vi "Cleanup Session.vi"(8 "error in":errorcluster, 11 "Plugin in":refnum<class "Power Spectrum Density.lvclass">) -> (0 "error out":errorcluster, 3 "Plugin out":refnum<class "Power Spectrum Density.lvclass">)   [LabVIEW 2023, in "Power Spectrum Density.lvlib" / "Power Spectrum Density.lvclass"]
uses:
  Power Spectrum Density.lvclass
  Buffer Manager Function.ctl
  Power Spectrum Density.lvclass/Power Spectrum Density.ctl
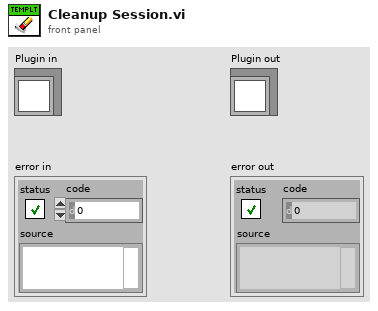
[diagram p1: front panel]
types:
  T1 = typedef "Power Spectrum Density.lvlib/Power Spectrum Density.lvclass/Buffer Manager Function.ctl" = enum16{"Get Data", "Buffer Data", "Reset Data"}
  T2 = enum32{"Invalid", "Standard", "Closed", "Hidden", "Minimized", "Maximized"}
  T3 = typedef "Power Spectrum Density.lvlib/Power Spectrum Density.lvclass/Power Spectrum Density Data.ctl" = cluster{"First Time":bool, "Show PSD Window":bool, "Show PSD Window Clicked":bool, "Export mode":T4, "Window":T5, "dB":bool, "Averaging parameters":cluster{"averaging mode":enum16{"No averaging", "Vector averaging", "RMS averaging", "Peak hold"}, "weighting mode":enum16{"Linear", "Exponential"}, "number of averages":u32}, "Window parameter":dbl, "Number of Samples":i32, "PSD VI Ref":refnum<vi>}
  T4 = typedef "NI_MAPro.lvlib/Power Spectrum and PSD Export Mode.ctl" = u16
  T5 = typedef "NI_AALPro.lvlib/windowTd.ctl" = u32
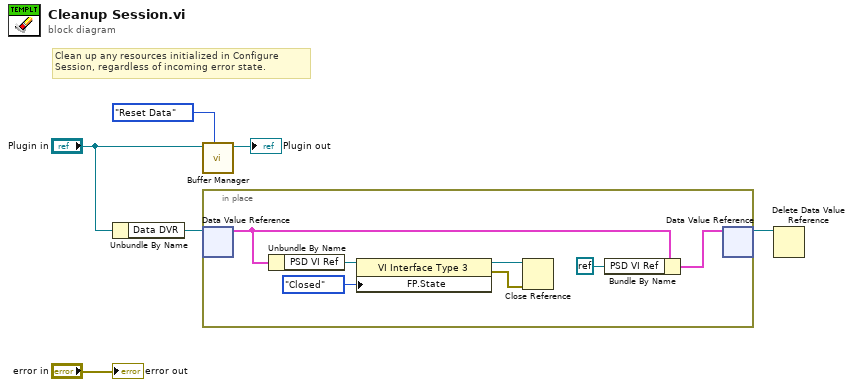
[diagram p0: block diagram]
diagram:
  # "Clean up any resources initialized in Configure Session, regardless of incoming error state."
  n1 = Unbundle By Name("Plugin in") -> ("Data DVR"=w6:refnum<data-value>)
  n2 = call-dynamic "Buffer Manager.vi"("Function"=Buffer_Manager_Function."Reset Data", "Plugin in"="Plugin in") -> ("Plugin out"=→"Plugin out":refnum<class "Power Spectrum Density.lvclass">)  [unwired: 5 in, 4 out]
  n3 = in-place {
    n4 = in-place-dvr #1(w6) -> (w13:T3)  [unwired: 1 out]
    n5 = Unbundle By Name(w13) -> ("PSD VI Ref"=w10:refnum<vi>)
    n6 = property class="VI Interface Type 3"(reference=w10, "FP.State"=T2."Closed" ("Front Panel Window:State")) -> (reference out=w9:refnum<vi>, error out=w7:errorcluster)  [unwired: 1 in]
    n7 = Close Reference(reference=w9, error in (no error)=w7) -> ()  [unwired: 1 out]
    n8 = Bundle By Name(cluster=w13, "PSD VI Ref"=refnum<k0> refnum) -> (w11:T3)
    n9 = in-place-dvr #1(w11) -> (w5:refnum<data-value>)  [unwired: 1 out]
  }
  n10 = Delete Data Value Reference(data value reference=w5) -> ()  [unwired: 1 in, 2 out]
  "error out" <- "error in"
